vi "testRegCmd.vi"(8 "error in (no error)":errorcluster) -> (0 "error out":errorcluster)   [LabVIEW 2018]
doc: "Test the regCmd.vi."
uses:
  src/TcpServer/TcpServer.lvclass
  src/TcpServer/TcpServer.lvclass/TcpServer.ctl
  src/TcpServerCmd/TcpServerCmd.lvclass/TcpServerCmd.ctl
  <vilib>/addons/_JKI Toolkits/Caraya/classes/Assert/Assert Equal Value_Variant.vi
  src/TcpServerCmd/TcpServerCmd.lvclass
  <vilib>/addons/_JKI Toolkits/Caraya/classes/Test/Test.lvclass
  <vilib>/addons/_JKI Toolkits/Caraya/classes/Assert/Assert.lvclass
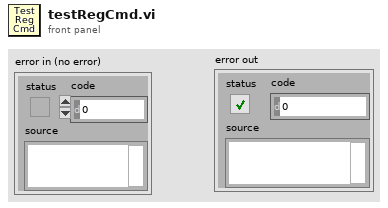
[diagram p1: front panel]
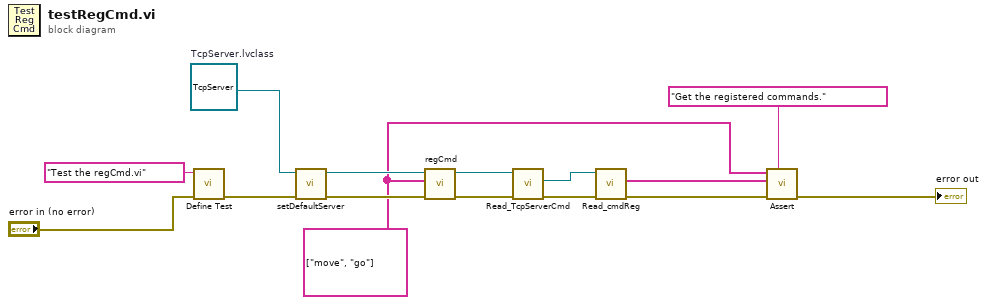
[diagram p0: block diagram]
diagram:
  w6 = string[] ["move", "go"] ("registeredCommands")
  w12 = refnum<class "TcpServer.lvclass"> refnum  # TcpServer.lvclass
  n1 = call <vilib>:"Define Test.vi"("error in (no error)"="error in (no error)", "Label (VI Title)"="Test the regCmd.vi") -> ("error out"=w14:errorcluster)  [unwired: 9 in]
  n2 = call "setDefaultServer.vi"("error in (no error)"=w14, "TcpServer.lvclass"=w12) -> ("error out"=w9:errorcluster, "tcpServer out"=w10:refnum<class "TcpServer.lvclass">)  [unwired: 8 in]
  n3 = call "regCmd.vi"("error in (no error)"=w9, "cmdReg"=w6, "tcpServer in"=w10) -> ("error out"=w4:errorcluster, "tcpServer out"=w2:refnum<class "TcpServer.lvclass">)  [unwired: 7 in]
  n4 = call "Read_TcpServerCmd.vi"("error in (no error)"=w4, "TcpServer in"=w2) -> ("error out"=w3:errorcluster, "TcpServerCmd.lvclass"=w1:refnum<class "TcpServerCmd.lvclass">)  [unwired: 7 in, 1 out]
  n5 = call "Read_cmdReg.vi"("error in (no error)"=w3, "TcpServerCmd in"=w1) -> ("error out"=w7:errorcluster, "cmdReg"=w5:string[])  [unwired: 7 in, 1 out]
  n6 = call-poly <vilib>:"Assert.vi"("Label"="Get the registered commands.", "error in (no error)"=w7, "Y"=w5, "X"=w6) -> ("error out"=→"error out":errorcluster)  [unwired: 7 in]
